vi "CRYCustom Editor.vi"() -> ()   [LabVIEW 2013]
uses:
  <vilib>/Utility/miscctls.llb/LVBoundsTypeDef.ctl
  Typedef Control/CRYCustom Cluster.ctl
  CRYProject/CRYProject Editor Global.vi
  CRYStepSetup/CRYStepSetup Global.vi
  CRYMainGlobal.vi
  CRYWindow/SubVI/CRYMain Sub Window Global.vi
panel:
  out "Custom":string
  out "Custom Bk":string
  in  "AddStep":bool
  in  "Add Lib":bool
  in  "stop":bool
  in  "Load Test":bool
  out "EndFlag":bool
  out "Proper VI No":i32
  in  "Save As":bool
  in  "Load":bool
  in  "Revert":bool
  out "VIMiniumBound":T1
  in  "Board Tab":enum32{"Page 1"}(tab) caption="Control Tab"
  in  "Cancel":bool caption="Apply"
  in  "OK":bool caption="Apply"
  in  "Sub Board Tab":enum32{"Setting", "Help"}(tab)
  out "Comment":bool
  in  "Unit":string caption="单位"
  in  "Byte":i32 caption="字节"
  in  "Curve Name":string caption="名称"
  in  "Select COM Port":i32(ring) caption="选择COM端口" items=["COM1", "COM2", "COM3", "COM4", "COM5", "COM6", "COM7", "COM8", "COM9", "COM10", "COM11", "COM12", "COM13", "COM14", "COM15", "COM16", "COM17", "COM18", "COM19", "COM20"]
  in  "Type":u16(ring) caption="类型" items=["从RS232读取在整数", "Sigma Extration", "系统", "你的步骤名称"]
  out "Reminder":bool
  in  "Help":string
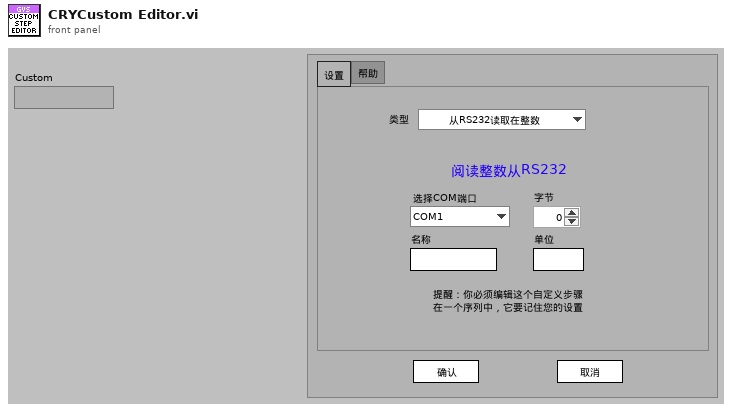
[diagram p1: front panel]
types:
  T1 = typedef "LVBoundsTypeDef.ctl" = cluster{"Width":u32, "Height":u32}
  T2 = cluster{"Type":u16, "Select COM Port":i32, "Byte":i32, "Unit":string, "Curve Name":string}
  T3 = typedef "CRYStep.ctl" = cluster{"No.VI":i32, "Category":string, "StepName":string, "Seq setup flattened":string, "Comment":string, "Steps config.":bool[], "Jump config":i32[], "Start":dbl, "Increment":dbl, "Name":string, "Unit":string, "Y data":u16, "Y prefix":string, "Y dB ref":dbl, "Y unit":string, "Repeat State Array":cluster{"Start":dbl, "Increment":dbl, "Count":i32, "Num":i32}[]}
  T4 = typedef "CRYCustom Cluster.ctl" = cluster{"Help":string, "Flatten Data":string}
  T5 = cluster{"Load Test":bool, "Add Lib":bool, "OK":bool, "Cancel":bool}
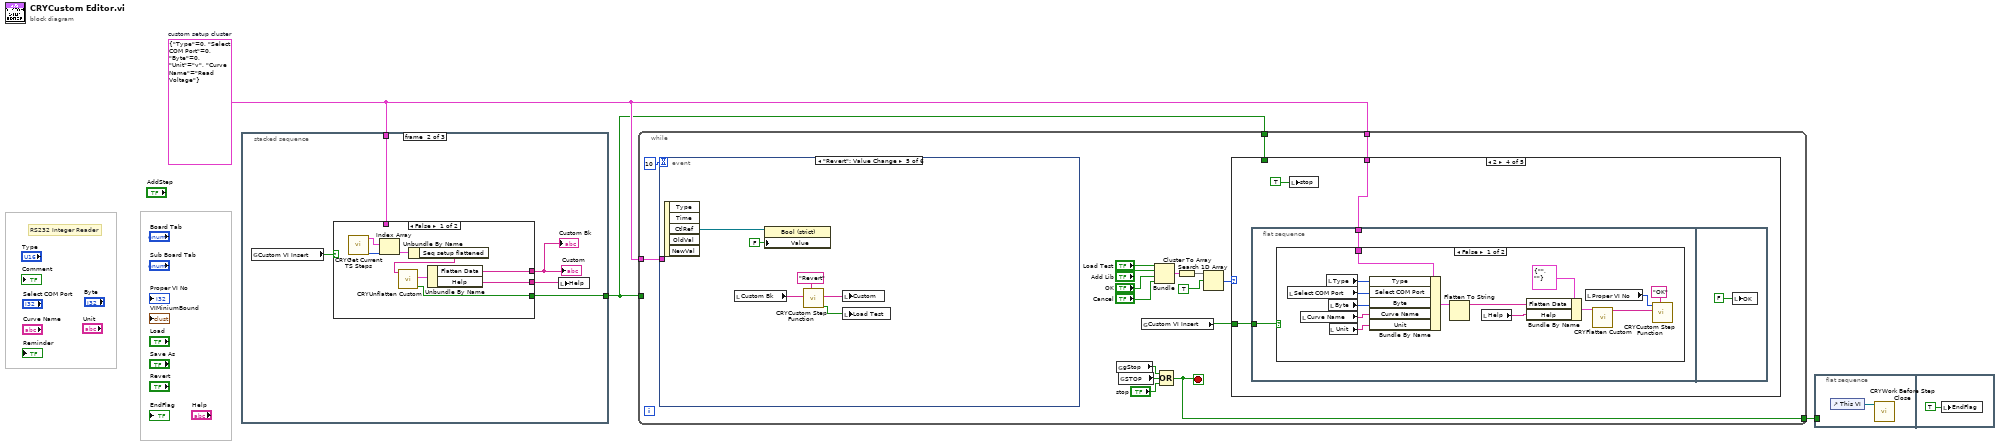
[diagram p0: block diagram]
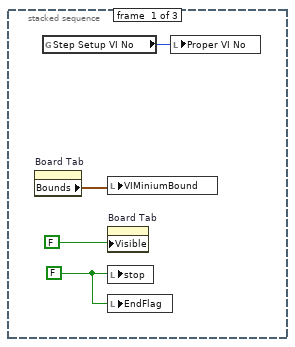
[diagram p2: hidden frame]
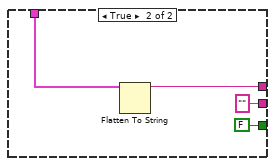
[diagram p3: hidden frame]
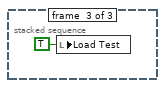
[diagram p4: hidden frame]
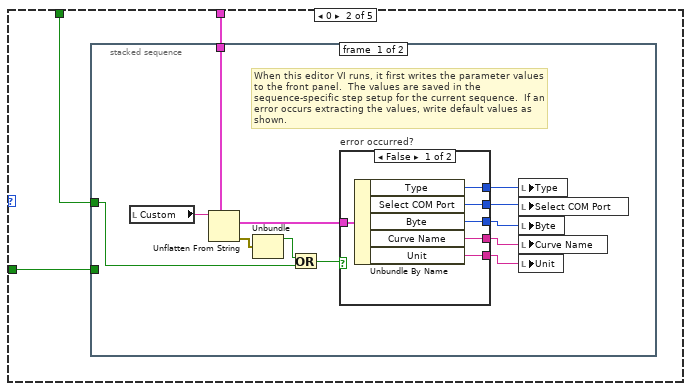
[diagram p6: hidden frame]
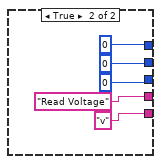
[diagram p7: hidden frame]
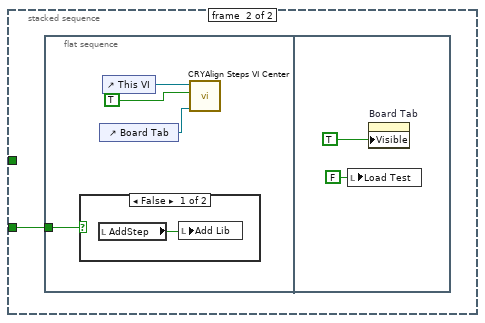
[diagram p8: hidden frame]
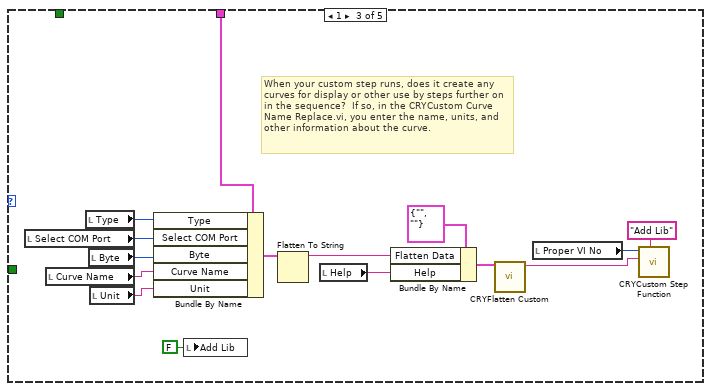
[diagram p10: hidden frame]
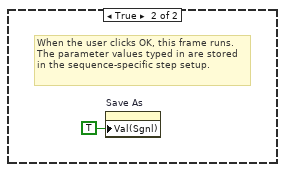
[diagram p11: hidden frame]
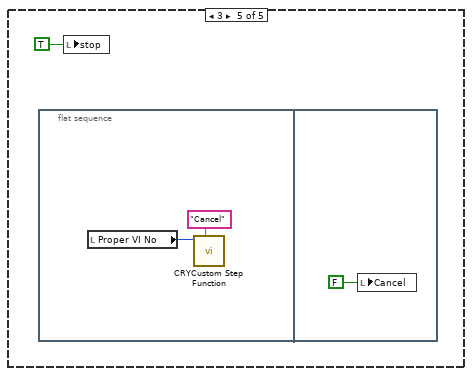
[diagram p12: hidden frame]
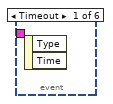
[diagram p13: hidden frame]
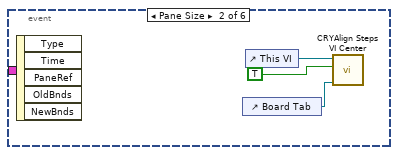
[diagram p14: hidden frame]
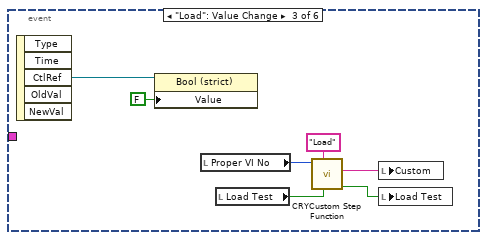
[diagram p15: hidden frame]
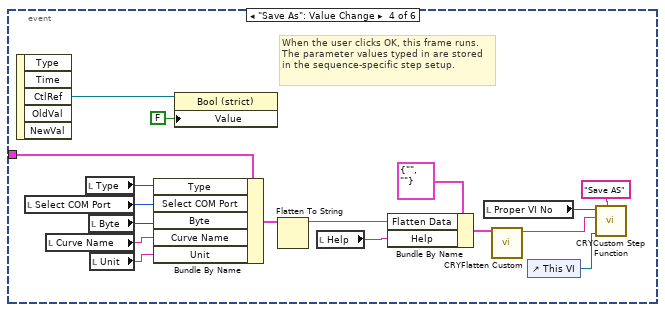
[diagram p16: hidden frame]
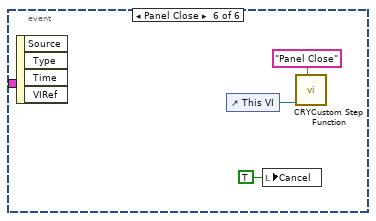
[diagram p17: hidden frame]
diagram:
  w2 = T2 {"Type"=0, "Select COM Port"=0, "Byte"=0, "Unit"="v", "Curve Name"="Read Voltage"}  # custom setup cluster
  # "RS232 Integer Reader"
  n1 = stacked-sequence {
    tunnel: w2 -> [_ w10 _]
    tunnel: [_ w9 _] -> w1
    frame #0 {
      w4 = FALSE ("stop")
      n2 = property on="Board Tab" class="TabCtl (strict)"() -> ("Bounds"=w7:T1)  [unwired: 2 in, 2 out]
      n3 = global read "CRYProject Editor Global.vi" "Step Setup VI No"() -> (w5:i32)
      n4 = local write "VIMiniumBound"(w7) -> ()
      n5 = property on="Board Tab" class="TabCtl (strict)"("Visible"=FALSE ("Load Test")) -> ()  [unwired: 2 in, 2 out]
      n6 = local write "stop"(w4) -> ()
      n7 = local write "EndFlag"(w4) -> ()
      n8 = local write "Proper VI No"(w5) -> ()
    }
    frame #1 {
      n9 = global read "CRYStepSetup Global.vi" "Custom VI Insert"() -> (w12:bool)
      n10 = case shown="False" w12 {
        tunnel: [w14 w23] -> w11
        tunnel: w10 -> [_ w24]
        tunnel: [w16 FALSE ("Error?")] -> w9
        tunnel: [w13 "" ("Help")] -> w8
        frame False {
          n11 = call "CRYGet Current TS Steps.vi"() -> ("SelectStepNumber in Tree"=w18:i32, "Steps"=w19:T3[])  [unwired: 7 in, 3 out]
          n12 = Index Array(array=w19, index=w18) -> (element=w20:T3)
          n13 = Unbundle By Name(w20) -> ("Seq setup flattened"=w15:string)
          n14 = call "CRYUnflatten Custom.vi"("Unflatten Custom"=w15) -> ("Error?"=w16:bool, "Custom"=w17:T4)  [unwired: 8 in, 1 out]
          n15 = Unbundle By Name(w17) -> ("Flatten Data"=w14:string, "Help"=w13:string)
        }
        frame True {
          n16 = Flatten To String(anything=w24) -> (data string=w23:string)  [unwired: 1 in, 4 out]
        }
      }
      "Custom" <- w11
      "Custom Bk" <- w11
      n17 = local write "Help"(w8) -> ()
    }
    frame #2 {
      n18 = local write "Load Test"(TRUE ("Load Test")) -> ()
    }
  }
  n19 = while {
    tunnel: [w33] -> w3
    tunnel: w2 -> [w28]
    tunnel: w2 -> [w27]
    tunnel: w1 -> [w26]
    tunnel: w1 -> [_]
    stop <- w33 stop-if-true
    n20 = event shown="[4] \"Revert\": Value Change" {
      selector: _ -> [_ _ _ _ _ _]
      dyn-events: _ -> [_ _ _ _ _ _]
      timeout: 10 -> [_ _ _ _ _ _]
      tunnel: w27 -> [_ _ _ w135 _ _]
      event Timeout {
        n21 = event-data() -> ()  [unwired: 1 in, 2 out]
      }
      event Pane Size {
        n22 = event-data() -> ()  [unwired: 1 in, 5 out]
        n23 = control-ref of="Board Tab"() -> (w117:refnum<vi>)
        n24 = control-ref of="This VI"() -> (w118:refnum<vi>)
        n25 = call "CRYAlign Steps VI Center.vi"("Tab2"=w117, "Input/Output"=TRUE ("Preview"), "VIRef"=w118) -> ()  [unwired: 1 in, 8 out]
      }
      event "Load": Value Change {
        n26 = event-data() -> ("CtlRef"=w125:refnum<vi>)  [unwired: 1 in, 4 out]
        n27 = property class="Bool (strict)"(reference=w125, "Value"=FALSE) -> ()  [unwired: 1 in, 2 out]
        n28 = local read "Proper VI No"() -> (w123:i32)
        n29 = local read "Load Test"() -> (w122:bool)
        n30 = call "CRYCustom Step Function.vi"("bData"=w122, "sAction"="Load" ("Action"), "nData"=w123) -> ("bData Out"=w120:bool, "sData Out"=w121:string)  [unwired: 7 in]
        n31 = local write "Custom"(w121) -> ()
        n32 = local write "Load Test"(w120) -> ()
      }
      event "Save As": Value Change {
        # "When the user clicks OK, this frame runs.  The parameter values typed in are stored in the sequence-specific step setup."
        n33 = event-data() -> ("CtlRef"=w142:refnum<vi>)  [unwired: 1 in, 4 out]
        n34 = local read "Select COM Port"() -> (w138:i32)
        n35 = local read "Curve Name"() -> (w140:string)
        n36 = local read "Type"() -> (w137:u16)
        n37 = local read "Byte"() -> (w139:i32)
        n38 = local read "Unit"() -> (w141:string)
        n39 = Bundle By Name(cluster=w135, "Type"=w137, "Select COM Port"=w138, "Byte"=w139, "Curve Name"=w140, "Unit"=w141) -> (w136:T2)
        n40 = property class="Bool (strict)"(reference=w142, "Value"=FALSE) -> ()  [unwired: 1 in, 2 out]
        n41 = Flatten To String(anything=w136) -> (data string=w131:string)  [unwired: 1 in, 4 out]
        n42 = local read "Help"() -> (w133:string)
        n43 = Bundle By Name(cluster=T4 {"Help"="", "Flatten Data"=""} ("Custom"), "Flatten Data"=w131, "Help"=w133) -> (w132:T4)
        n44 = local read "Proper VI No"() -> (w128:i32)
        n45 = call "CRYFlatten Custom.vi"("Custom"=w132) -> ("Flatten Custom String"=w127:string)  [unwired: 10 in]
        n46 = control-ref of="This VI"() -> (w129:refnum<vi>)
        n47 = call "CRYCustom Step Function.vi"("sAction"="Save AS" ("Action"), "VI Ref"=w129, "sData"=w127, "nData"=w128) -> ()  [unwired: 6 in, 2 out]
      }
      event "Revert": Value Change {
        n48 = event-data() -> ("CtlRef"=w149:refnum<vi>)  [unwired: 1 in, 4 out]
        n49 = local read "Custom Bk"() -> (w144:string)
        n50 = property class="Bool (strict)"(reference=w149, "Value"=FALSE) -> ()  [unwired: 1 in, 2 out]
        n51 = call "CRYCustom Step Function.vi"("sAction"="Revert" ("Action"), "sData"=w144) -> ("bData Out"=w146:bool, "sData Out"=w145:string)  [unwired: 8 in]
        n52 = local write "Custom"(w145) -> ()
        n53 = local write "Load Test"(w146) -> ()
      }
      event Panel Close {
        n54 = event-data() -> ()  [unwired: 1 in, 4 out]
        n55 = control-ref of="This VI"() -> (w150:refnum<vi>)
        n56 = local write "Cancel"(TRUE ("Cancel")) -> ()
        n57 = call "CRYCustom Step Function.vi"("sAction"="Panel Close" ("Action"), "VI Ref"=w150) -> ()  [unwired: 8 in, 2 out]
      }
    }
    n58 = global read "CRYMain Sub Window Global.vi" "gStop"() -> (w36:bool)
    n59 = global read "CRYMainGlobal.vi" "STOP"() -> (w34:bool)
    n60 = global read "CRYStepSetup Global.vi" "Custom VI Insert"() -> (w29:bool)
    n61 = Bundle("Load Test"="Load Test", "Add Lib"="Add Lib", "OK"="OK", "Cancel"="Cancel") -> (w40:T5)  [unwired: 1 out]
    n62 = Compound Arithmetic op=OR(w36, w34, "stop") -> (w33:bool)
    n63 = Cluster To Array(cluster=w40) -> (array=w39:bool[])
    n64 = Search 1D Array(1D array=w39, element=TRUE) -> (index of element=w37:i32)  [unwired: 1 out]
    n65 = case shown="2" w37 {
      tunnel: w29 -> [_ w45 _ w93 _]
      tunnel: w28 -> [_ w44 w84 w92 _]
      tunnel: w26 -> [_ w43 _ _ _]
      frame Default {
      }
      frame 0 {
        n66 = stacked-sequence {
          tunnel: w45 -> [_ w69]
          tunnel: w44 -> [w53 _]
          tunnel: w43 -> [w46 _]
          frame #0 {
            # "When this editor VI runs, it first writes the parameter values to the front panel.  The values are saved in the sequence-specific step setup for the current sequence.  If an error occurs extracting the values, write default values as shown."
            n67 = local read "Custom"() -> (w47:string)
            n68 = Unflatten From String(type=w53, binary string=w47) -> (value=w56:T2, error out=w57:errorcluster)  [unwired: 1 in, 3 out]
            n69 = Unbundle(w57) -> ("status"=w54:bool)  [unwired: 2 out]
            n70 = Or(x=w54, y=w46) -> (x .or. y?=w55:bool)
            n71 = case "error occurred?" shown="False" w55 {
              tunnel: w56 -> [w63 _]
              tunnel: [w62 0 ("Select COM Port")] -> w51
              tunnel: [w61 u16 0 ("Type")] -> w52
              tunnel: [w60 0 ("Byte")] -> w50
              tunnel: [w59 "Read Voltage" ("Curve Name")] -> w49
              tunnel: [w58 "v" ("Unit")] -> w48
              frame False {
                n72 = Unbundle By Name(w63) -> ("Type"=w61:u16, "Select COM Port"=w62:i32, "Byte"=w60:i32, "Curve Name"=w59:string, "Unit"=w58:string)
              }
              frame True {
              }
            }
            n73 = local write "Type"(w52) -> ()
            n74 = local write "Select COM Port"(w51) -> ()
            n75 = local write "Byte"(w50) -> ()
            n76 = local write "Curve Name"(w49) -> ()
            n77 = local write "Unit"(w48) -> ()
          }
          frame #1 {
            n78 = flat-sequence {
              tunnel: w69 -> [w70]
              frame #0 {
                n79 = case shown="False" w70 {
                  frame False {
                    n80 = local read "AddStep"() -> (w74:bool)
                    n81 = local write "Add Lib"(w74) -> ()
                  }
                  frame True {
                  }
                }
                n82 = control-ref of="Board Tab"() -> (w71:refnum<vi>)
                n83 = control-ref of="This VI"() -> (w72:refnum<vi>)
                n84 = call "CRYAlign Steps VI Center.vi"("Tab2"=w71, "Input/Output"=TRUE ("Preview"), "VIRef"=w72) -> ()  [unwired: 1 in, 8 out]
              }
              frame #1 {
                n85 = local write "Load Test"(FALSE ("Load Test")) -> ()
                n86 = property on="Board Tab" class="TabCtl (strict)"("Visible"=TRUE ("Load Test")) -> ()  [unwired: 2 in, 2 out]
              }
            }
          }
        }
      }
      frame 1 {
        # "When your custom step runs, does it create any curves for display or other use by steps further on in the sequence?  If so, in the CRYCustom Curve Name Replace.vi, you enter the name, units, and other information about the curve."
        n87 = local read "Select COM Port"() -> (w87:i32)
        n88 = local read "Curve Name"() -> (w89:string)
        n89 = local read "Type"() -> (w86:u16)
        n90 = local read "Byte"() -> (w88:i32)
        n91 = local read "Unit"() -> (w90:string)
        n92 = Bundle By Name(cluster=w84, "Type"=w86, "Select COM Port"=w87, "Byte"=w88, "Curve Name"=w89, "Unit"=w90) -> (w85:T2)
        n93 = local write "Add Lib"(FALSE ("Add Lib")) -> ()
        n94 = Flatten To String(anything=w85) -> (data string=w80:string)  [unwired: 1 in, 4 out]
        n95 = local read "Help"() -> (w82:string)
        n96 = Bundle By Name(cluster=T4 {"Help"="", "Flatten Data"=""} ("Custom"), "Flatten Data"=w80, "Help"=w82) -> (w83:T4)
        n97 = call "CRYFlatten Custom.vi"("Custom"=w83) -> ("Flatten Custom String"=w77:string)  [unwired: 10 in]
        n98 = local read "Proper VI No"() -> (w79:i32)
        n99 = call "CRYCustom Step Function.vi"("sAction"="Add Lib" ("Action"), "sData"=w77, "nData"=w79) -> ()  [unwired: 7 in, 2 out]
      }
      frame 2 {
        n100 = flat-sequence {
          tunnel: w93 -> [w96]
          tunnel: w92 -> [w95]
          frame #0 {
            n101 = case shown="False" w96 {
              tunnel: w95 -> [w110 _]
              frame False {
                n102 = local read "Select COM Port"() -> (w107:i32)
                n103 = local read "Curve Name"() -> (w105:string)
                n104 = local read "Type"() -> (w108:u16)
                n105 = local read "Byte"() -> (w106:i32)
                n106 = local read "Unit"() -> (w104:string)
                n107 = Bundle By Name(cluster=w110, "Type"=w108, "Select COM Port"=w107, "Byte"=w106, "Curve Name"=w105, "Unit"=w104) -> (w109:T2)
                n108 = Flatten To String(anything=w109) -> (data string=w99:string)  [unwired: 1 in, 4 out]
                n109 = local read "Help"() -> (w101:string)
                n110 = Bundle By Name(cluster=T4 {"Help"="", "Flatten Data"=""} ("Custom"), "Flatten Data"=w99, "Help"=w101) -> (w100:T4)
                n111 = local read "Proper VI No"() -> (w103:i32)
                n112 = call "CRYFlatten Custom.vi"("Custom"=w100) -> ("Flatten Custom String"=w98:string)  [unwired: 10 in]
                n113 = call "CRYCustom Step Function.vi"("sAction"="OK" ("Action"), "sData"=w98, "nData"=w103) -> ()  [unwired: 7 in, 2 out]
              }
              frame True {
                # "When the user clicks OK, this frame runs.  The parameter values typed in are stored in the sequence-specific step setup."
                n114 = property on="Save As" class="Bool (strict)"("Val(Sgnl)"=TRUE ("Value (Signaling)")) -> ()  [unwired: 2 in, 2 out]
              }
            }
          }
          frame #1 {
            n115 = local write "OK"(FALSE ("OK")) -> ()
          }
        }
        n116 = local write "stop"(TRUE ("stop")) -> ()
      }
      frame 3 {
        n117 = flat-sequence {
          frame #0 {
            n118 = local read "Proper VI No"() -> (w114:i32)
            n119 = call "CRYCustom Step Function.vi"("sAction"="Cancel" ("Action"), "nData"=w114) -> ()  [unwired: 8 in, 2 out]
          }
          frame #1 {
            n120 = local write "Cancel"(FALSE ("Cancel")) -> ()
          }
        }
        n121 = local write "stop"(TRUE ("stop")) -> ()
      }
    }
  }
  n122 = flat-sequence {
    tunnel: w3 -> [_]
    frame #0 {
      n123 = control-ref of="This VI"() -> (w153:refnum<vi>)
      n124 = call "CRYWork Before Step Close.vi"("StepVI Ref"=w153) -> ()  [unwired: 11 in]
    }
    frame #1 {
      n125 = local write "EndFlag"(TRUE ("EndFlag")) -> ()
    }
  }
